vi "Add Relay Suffix.vi"(8 "topology suffix":string, 10 "Relays":string[](array[string])) -> (1 "Array":string[](array[string]))   [LabVIEW 2015, in "SLSC Switch.lvlib" / "SLSC Switch.lvclass"]
uses:
  SLSC Switch.lvclass
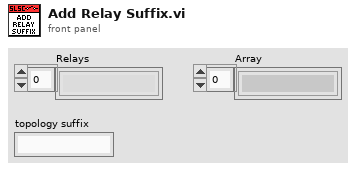
[diagram p1: front panel]
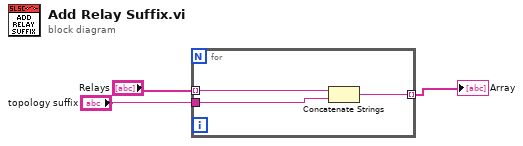
[diagram p0: block diagram]
diagram:
  n1 = for {
    tunnel: "Relays" -> [w6] mode=indexing
    tunnel: "topology suffix" -> [w5]
    tunnel: [w4] -> w3 mode=indexing
    n2 = Concatenate Strings(w6, w5) -> (w4:string)
  }
  "Array" <- w3
